vi "MeasureSTARTTime.vi"(8 "error in":errorcluster, 11 "VISA resource name":refnum<visa-resource-name>) -> (0 "error out":errorcluster, 2 "System time":dbl=437416.625 format="%.3f", 3 "VISA resource name out":refnum<visa-resource-name>)   [LabVIEW 2018, in "GP22_TDC_Arduinoed.lvlib"]
doc: "Measure the time of arrival of the next pulse at the START input, in milliseconds since the unit was last reset. The counter rolls over every 24 hours."
uses:
  GP22_TDC_Arduinoed.lvlib
  <vilib>/Utility/error.llb/Error Cluster From Error Code.vi
  <vilib>/regexp/Match Regular Expression.xnode
  <vilib>/ErrorRing/Error Ring.xnode
panel:
  in  "Timeout / ms":u32=1000
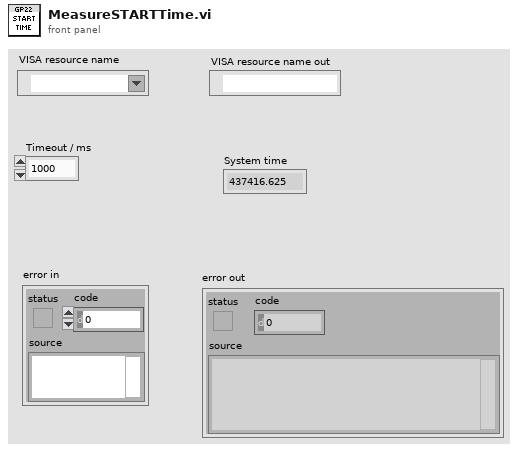
[diagram p1: front panel]
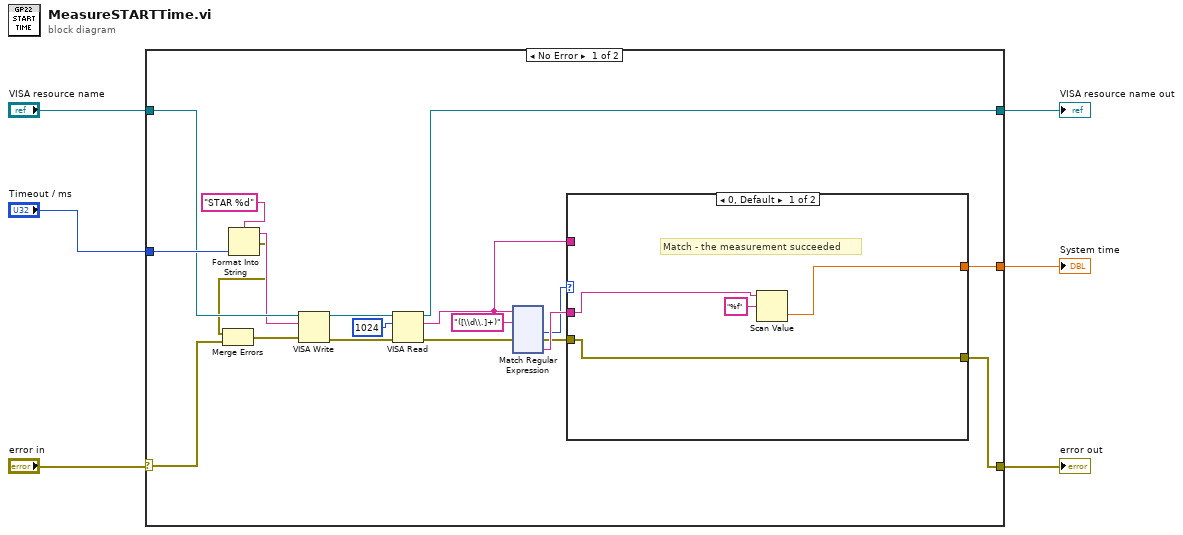
[diagram p0: block diagram]
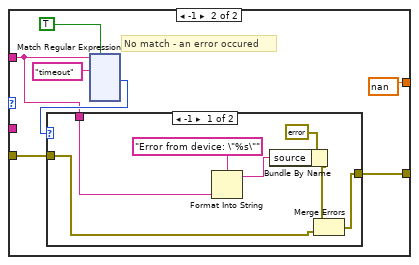
[diagram p2: hidden frame]
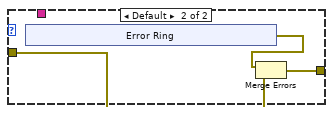
[diagram p3: hidden frame]
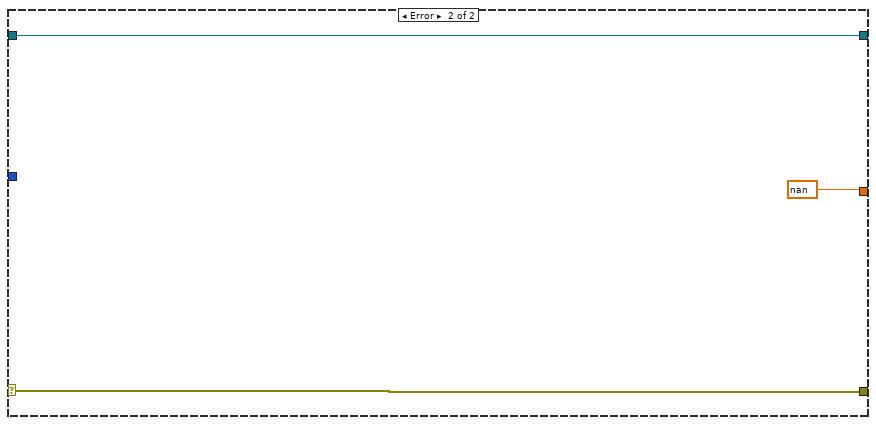
[diagram p4: hidden frame]
diagram:
  n1 = case shown="No Error" "error in" {
    selector: "error in" -> [w19 w286]
    tunnel: "VISA resource name" -> [w23 w285]
    tunnel: [w15 w285] -> w5
    tunnel: [w14 w286] -> w4
    tunnel: "Timeout / ms" -> [w24 _]
    tunnel: [w13 nan] -> w1
    frame No Error {
      n2 = Format Into String(format string="STAR %d", w24) -> (resulting string=w22:string, error out=w20:errorcluster)  [unwired: 2 in]
      n3 = Merge Errors(w20, w19) -> (w21:errorcluster)
      n4 = VISA Write(VISA resource name=w23, write buffer=w22, error in (no error)=w21) -> (VISA resource name out=w17:refnum<visa-resource-name>, error out=w18:errorcluster)  [unwired: 1 out]
      n5 = VISA Read(VISA resource name=w17, byte count=u32 1024, error in (no error)=w18) -> (VISA resource name out=w15:refnum<visa-resource-name>, read buffer=w7:string, error out=w11:errorcluster)  [unwired: 1 out]
      n6 = xnode "Match Regular Expression"("input string"=w7, "regular expression"="([\\d\\.]+)", "error in"=w11) -> ("offset past match"=w9:i32, "error out"=w8:errorcluster, "submatch 1"=w10:string)  [unwired: 3 in, 3 out]
      n7 = case shown="0, Default" w9 {
        tunnel: w8 -> [w142 w151]
        tunnel: [w142 w152] -> w14
        tunnel: w10 -> [w144 _]
        tunnel: [w143 nan] -> w13
        tunnel: w7 -> [_ w146]
        frame 0, Default {
          # "Match - the measurement succeeded"
          n8 = Scan Value(string=w144, format string="%f") -> (value=w143:dbl)  [unwired: 1 in, 1 out]
        }
        frame -1 {
          # "No match - an error occured"
          n9 = xnode "Match Regular Expression"("input string"=w146, "regular expression"="timeout", "ignore case? (F)"=TRUE) -> ("offset past match"=w147:i32)  [unwired: 3 in, 5 out]
          n10 = case shown="-1" w147 {
            tunnel: [w156 w162] -> w152
            tunnel: w151 -> [w155 w160]
            tunnel: w146 -> [w153 _]
            frame -1 {
              n11 = Format Into String(format string="Error from device: \"%s\"", w153) -> (resulting string=w158:string)  [unwired: 2 in, 1 out]
              n12 = Bundle By Name(cluster=errorcluster {"status"=TRUE, "code"=5000, "source"=""} ("error constant"), "source"=w158) -> (w157:errorcluster)
              n13 = Merge Errors(w157, w155) -> (w156:errorcluster)
            }
            frame Default {
              n14 = xnode "Error Ring"() -> ("error out"=w161:errorcluster)
              n15 = Merge Errors(w161, w160) -> (w162:errorcluster)
            }
          }
        }
      }
    }
    frame Error {
    }
  }
  "VISA resource name out" <- w5
  "error out" <- w4
  "System time" <- w1
